vi "Ex4.vi"() -> ()   [LabVIEW 2012]
uses:
  <userlib>/ROSforLV/ROS/Code/JointPositions.ctl
  <userlib>/ROSforLV/ROS/Code/Slider.ctl
panel:
  in  "Bring Arms In":bool
  in  "Reset to Zero":bool
  in  "Joint Positions":T1 {"left_w2" scale=-180.0..180.0; "left_w1" scale=-180.0..180.0; "left_w0" scale=-180.0..180.0; "left_e1" scale=-180.0..180.0; "left_e0" scale=-180.0..180.0; "left_s1" scale=-180.0..180.0; "left_s0" scale=-180.0..180.0; "right_s1" scale=-180.0..180.0; "right_s0" scale=-180.0..180.0; "right_w2" scale=-180.0..180.0; "right_e1" scale=-180.0..180.0; "right_e0" scale=-180.0..180.0; "right_w0" scale=-180.0..180.0; "right_w1" scale=-180.0..180.0}
  in  "stop":bool
  # "Control Baxter's Arms using the supplied Position Controller"
  # "Currently fails to open /robot/limb/right/command_joint_angles due to issue 2 - Multiple Publishers in Loop \n(https://github.com/chris-smith/ROSforLabview/issues/2)"
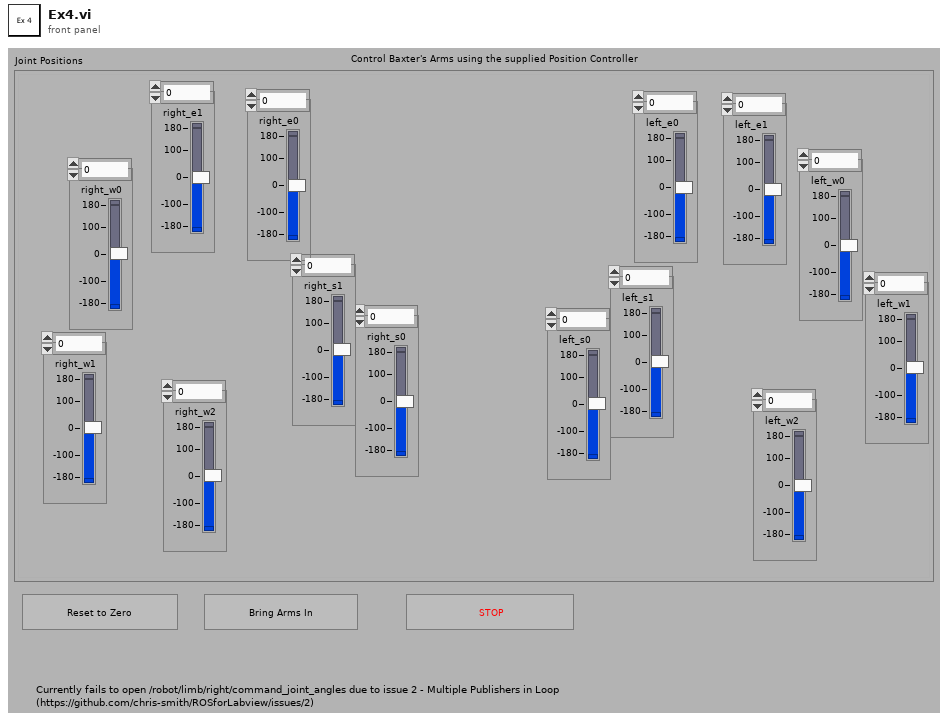
[diagram p1: front panel]
types:
  T1 = typedef "JointPositions.ctl" = cluster{"left_e0":T2, "left_e1":T2, "left_s0":T2, "left_s1":T2, "left_w0":T2, "left_w1":T2, "left_w2":T2, "right_e0":T2, "right_e1":T2, "right_s0":T2, "right_s1":T2, "right_w0":T2, "right_w1":T2, "right_w2":T2}
  T2 = typedef "Slider.ctl" = dbl
  T3 = cluster{"Joint Name":string, "Position":dbl, "Velocity":dbl, "Effort":dbl}[]
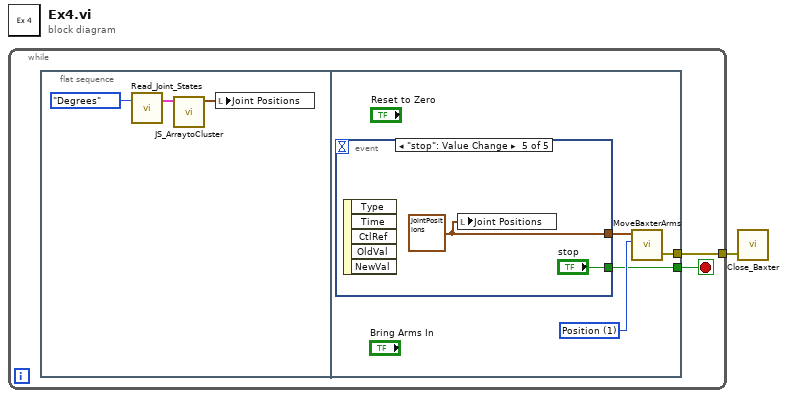
[diagram p0: block diagram]
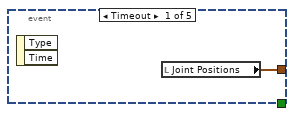
[diagram p2: hidden frame]
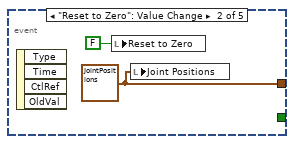
[diagram p3: hidden frame]
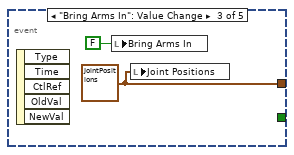
[diagram p4: hidden frame]
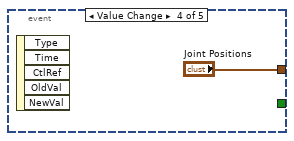
[diagram p5: hidden frame]
diagram:
  n1 = while {
    tunnel: [w3] -> w1
    stop <- w2 stop-if-true
    n2 = flat-sequence {
      tunnel: [w10] -> w3
      tunnel: [w7] -> w2
      frame #0 {
        n3 = call <userlib>:"Read_Joint_States.vi"("Units (deg)"=enum16{"Radians", "Degrees"}."Degrees") -> ("Joint States"=w6:T3)  [unwired: 2 in, 1 out]
        n4 = call <userlib>:"JS_ArraytoCluster.vi"("Joint States"=w6) -> ("Joint Positions 2"=w5:T1)  [unwired: 10 in]
        n5 = local write "Joint Positions"(w5) -> ()
      }
      frame #1 {
        w9 = u8 1 items=["Position"=1, "Velocity"=2, "Effort"=3] ("Mode")
        n6 = event shown="[4] \"stop\": Value Change" {
          selector: _ -> [_ _ _ _ _]
          dyn-events: _ -> [_ _ _ _ _]
          timeout: _ -> [_ _ _ _ _]
          tunnel: [w11 w12 w14 "Joint Positions" w17] -> w8
          tunnel: [_ _ _ _ "stop"] -> w7
          event Timeout {
            n7 = event-data() -> ()  [unwired: 1 in, 2 out]
            n8 = local read "Joint Positions"() -> (w11:T1)
          }
          event "Reset to Zero": Value Change {
            w12 = T1 {"left_e0"=0.0, "left_e1"=0.0, "left_s0"=0.0, "left_s1"=0.0, "left_w0"=0.0, "left_w1"=0.0, "left_w2"=0.0, "right_e0"=0.0, "right_e1"=0.0, "right_s0"=0.0, "right_s1"=0.0, "right_w0"=0.0, "right_w1"=0.0, "right_w2"=0.0} ("Joint Positions 2")
            n9 = event-data() -> ()  [unwired: 1 in, 4 out]
            n10 = local write "Reset to Zero"(FALSE ("Reset to Zero")) -> ()
            n11 = local write "Joint Positions"(w12) -> ()
          }
          event "Bring Arms In": Value Change {
            w14 = T1 {"left_e0"=0.0, "left_e1"=90.0, "left_s0"=-30.0, "left_s1"=0.0, "left_w0"=0.0, "left_w1"=0.0, "left_w2"=0.0, "right_e0"=0.0, "right_e1"=90.0, "right_s0"=30.0, "right_s1"=0.0, "right_w0"=0.0, "right_w1"=0.0, "right_w2"=0.0} ("Joint Positions 2")
            n12 = event-data() -> ()  [unwired: 1 in, 5 out]
            n13 = local write "Bring Arms In"(FALSE ("Bring Arms In")) -> ()
            n14 = local write "Joint Positions"(w14) -> ()
          }
          event Value Change {
            n15 = event-data() -> ()  [unwired: 1 in, 5 out]
          }
          event "stop": Value Change {
            w17 = T1 {"left_e0"=0.0, "left_e1"=90.0, "left_s0"=-30.0, "left_s1"=0.0, "left_w0"=0.0, "left_w1"=0.0, "left_w2"=0.0, "right_e0"=0.0, "right_e1"=90.0, "right_s0"=30.0, "right_s1"=0.0, "right_w0"=0.0, "right_w1"=0.0, "right_w2"=0.0} ("Joint Positions 2")
            n16 = event-data() -> ()  [unwired: 1 in, 5 out]
            n17 = local write "Joint Positions"(w17) -> ()
          }
        }
        n18 = call <userlib>:"MoveBaxterArms.vi"("Parameters"=w8, "Mode"=w9) -> ("error out"=w10:errorcluster)  [unwired: 4 in]
      }
    }
  }
  n19 = call <userlib>:"Close_Baxter.vi"("error in"=w1) -> ()  [unwired: 3 in, 1 out]
